vi "ZeroMQ_TCS.vi"() -> ()   [LabVIEW 2018]
uses:
  <vilib>/addons/zeromq/socket_type.ctl
  <vilib>/addons/zeromq/socket_options.ctl
  <vilib>/addons/zeromq/zeromq.lvlib
  <vilib>/addons/zeromq/zmq_socket.lvclass
  <vilib>/addons/zeromq/zmq_context.lvclass
panel:
  in  "stop 3":bool
  out "command":string
  out "error out 3":errorcluster
  out "message":string
  out "error out 2":errorcluster
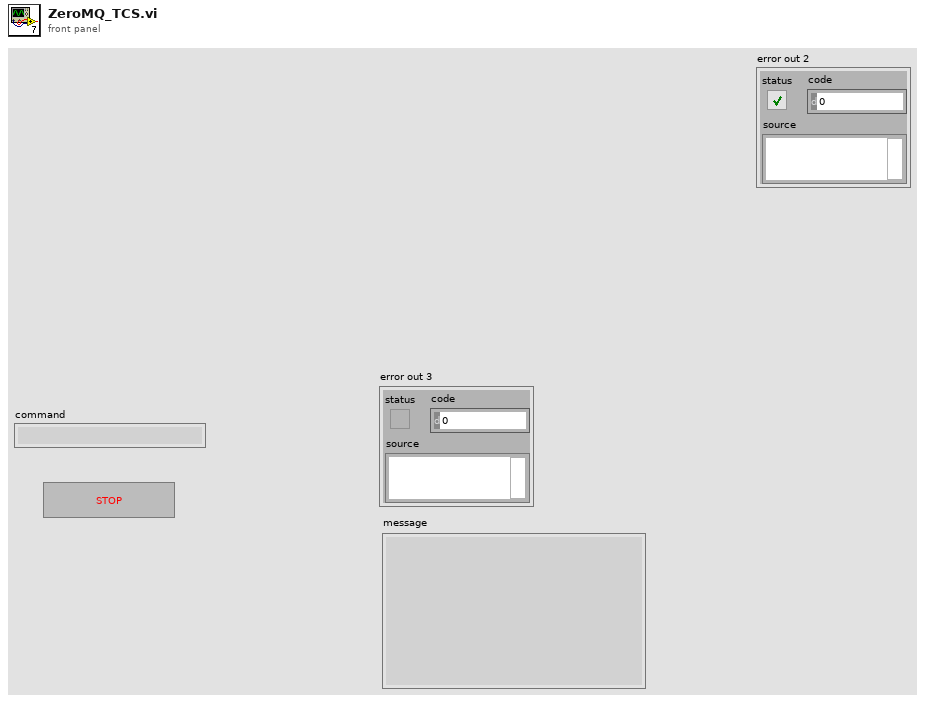
[diagram p1: front panel]
types:
  T1 = cluster{"ID":u32, "Address":string, "Service Name 1":string, "Service Name 2":string, "queue TX":refnum<queue>, "queue RX":refnum<queue>, "Port 1":u32, "Port 2":u32}
  T2 = typedef "zeromq.lvlib/socket_options.ctl" = enum8{"NONE", "ZMQ_HWM", "<2>", "ZMQ_SWAP", "ZMQ_AFFINITY", "ZMQ_ROUTING_ID", "ZMQ_SUBSCRIBE", "ZMQ_UNSUBSCRIBE", "ZMQ_RATE", "ZMQ_RECOVERY_IVL", "ZMQ_MCAST_LOOP", "ZMQ_SNDBUF", "ZMQ_RCVBUF", "ZMQ_RCVMORE", "ZMQ_FD", "ZMQ_EVENTS", "ZMQ_TYPE", "ZMQ_LINGER", "ZMQ_RECONNECT_IVL", "ZMQ_BACKLOG", "ZMQ_RECOVERY_IVL_MSEC", "ZMQ_RECONNECT_IVL_MAX", "ZMQ_MAXMSGSIZE", "ZMQ_SNDHWM", "ZMQ_RCVHWM", "ZMQ_MULTICAST_HOPS", "<26>", "ZMQ_RCVTIMEO", "ZMQ_SNDTIMEO", "<29>", "<30>", "ZMQ_IPV4ONLY", "ZMQ_LAST_ENDPOINT", "ZMQ_ROUTER_MANDATORY", "ZMQ_TCP_KEEPALIVE", "ZMQ_TCP_KEEPALIVE_CNT", "ZMQ_TCP_KEEPALIVE_IDLE", "ZMQ_TCP_KEEPALIVE_INTVL", "ZMQ_TCP_ACCEPT_FILTER", "ZMQ_IMMEDIATE", "ZMQ_XPUB_VERBOSE", "ZMQ_ROUTER_RAW", "ZMQ_IPV6", "ZMQ_MECHANISM", "ZMQ_PLAIN_SERVER", "ZMQ_PLAIN_USERNAME", "ZMQ_PLAIN_PASSWORD", "ZMQ_CURVE_SERVER", "ZMQ_CURVE_PUBLICKEY", "ZMQ_CURVE_SECRETKEY", "ZMQ_CURVE_SERVERKEY", "ZMQ_PROBE_ROUTER", "ZMQ_REQ_CORRELATE", "ZMQ_REQ_RELAXED", "ZMQ_CONFLATE", "ZMQ_ZAP_DOMAIN", "ZMQ_ROUTER_HANDOVER", "ZMQ_TOS", "ZMQ_IPC_FILTER_PID", "ZMQ_IPC_FILTER_UID", "ZMQ_IPC_FILTER_GID", "ZMQ_CONNECT_ROUTING_ID", "ZMQ_GSSAPI_SERVER", "ZMQ_GSSAPI_PRINCIPAL", "ZMQ_GSSAPI_SERVICE_PRINCIPAL", "ZMQ_GSSAPI_PLAINTEXT", "ZMQ_HANDSHAKE_IVL", "<67>", "ZMQ_SOCKS_PROXY", "ZMQ_XPUB_NODROP", "ZMQ_BLOCKY", "ZMQ_XPUB_MANUAL", "ZMQ_XPUB_WELCOME_MSG", "ZMQ_STREAM_NOTIFY", "ZMQ_INVERT_MATCHING", "ZMQ_HEARTBEAT_IVL", "ZMQ_HEARTBEAT_TTL", "ZMQ_HEARTBEAT_TIMEOUT", "ZMQ_XPUB_VERBOSER", "ZMQ_CONNECT_TIMEOUT", "ZMQ_TCP_MAXRT", "ZMQ_THREAD_SAFE", "<82>", "<83>", "ZMQ_MULTICAST_MAXTPDU", "ZMQ_VMCI_BUFFER_SIZE", "ZMQ_VMCI_BUFFER_MIN_SIZE", "ZMQ_VMCI_BUFFER_MAX_SIZE", "ZMQ_VMCI_CONNECT_TIMEOUT", "ZMQ_USE_FD", "ZMQ_GSSAPI_PRINCIPAL_NAMETYPE", "ZMQ_GSSAPI_SERVICE_PRINCIPAL_NAMETYPE", "ZMQ_BINDTODEVICE", "ZMQ_ZAP_ENFORCE_DOMAIN", "ZMQ_LOOPBACK_FASTPATH", "ZMQ_METADATA", "ZMQ_MULTICAST_LOOP", "ZMQ_ROUTER_NOTIFY"}
  T3 = typedef "zeromq.lvlib/socket_type.ctl" = enum8{"ZMQ_PAIR", "ZMQ_PUB", "ZMQ_SUB", "ZMQ_REQ", "ZMQ_REP", "ZMQ_DEALER", "ZMQ_ROUTER", "ZMQ_PULL", "ZMQ_PUSH", "ZMQ_XPUB", "ZMQ_XSUB", "ZMQ_STREAM", "ZMQ_SERVER", "ZMQ_CLIENT", "ZMQ_RADIO", "ZMQ_DISH", "ZMQ_GATHER", "ZMQ_SCATTER", "ZMQ_DGRAM"}
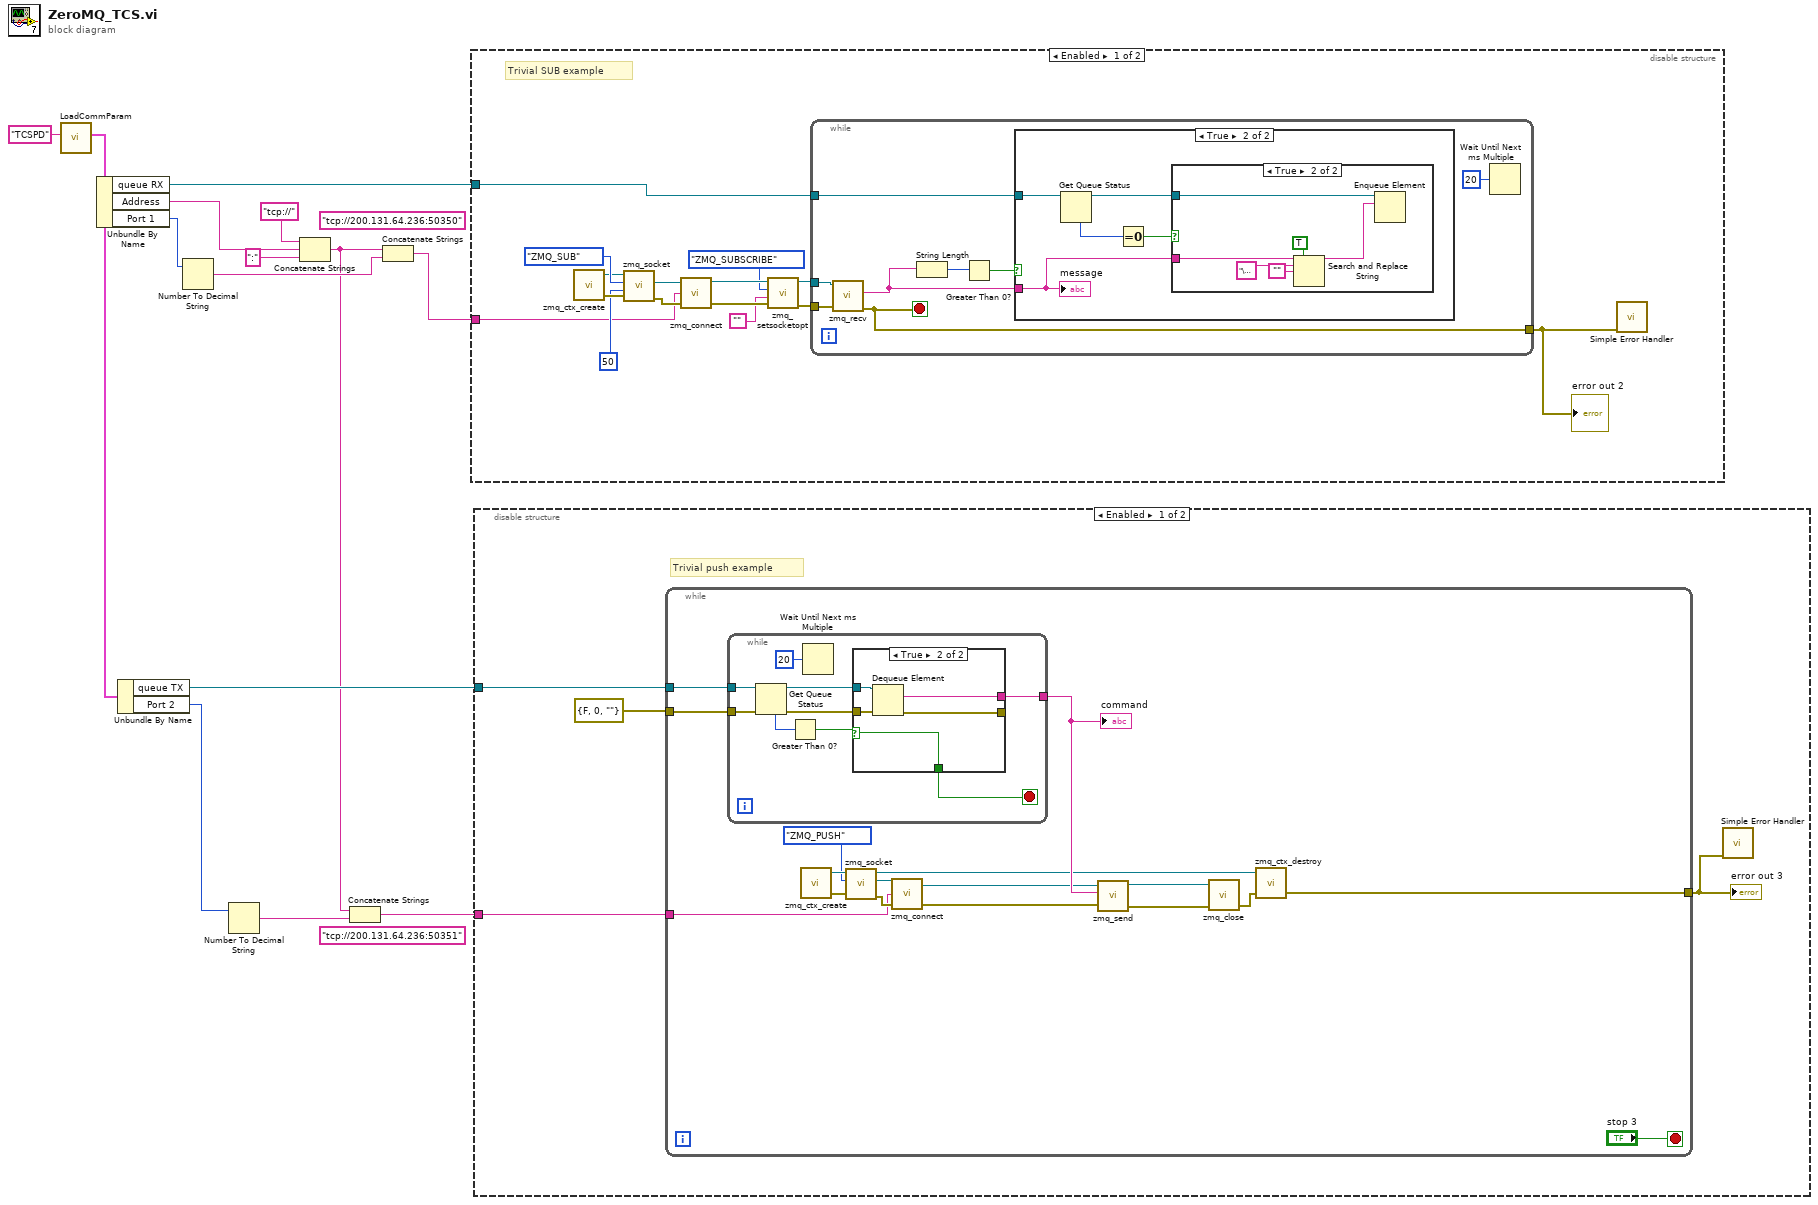
[diagram p0: block diagram]
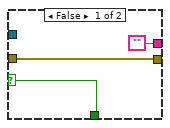
[diagram p2: hidden frame]
diagram:
  (unwired) "tcp://200.131.64.236:50351" ("endpoint")
  (unwired) "tcp://200.131.64.236:50350" ("endpoint")
  n1 = call "LoadCommParam.vi"("section name"="TCSPD") -> ("output cluster"=w7:T1)  [unwired: 10 in]
  n2 = Unbundle By Name(w7) -> ("queue RX"=w13:refnum<queue>, "Address"=w11:string, "Port 1"=w9:u32)
  n3 = Unbundle By Name(w7) -> ("queue TX"=w8:refnum<queue>, "Port 2"=w4:u32)
  n4 = Number To Decimal String(number=w9) -> (decimal integer string=w6:string)  [unwired: 1 in]
  n5 = Number To Decimal String(number=w4) -> (decimal integer string=w2:string)  [unwired: 1 in]
  n6 = Concatenate Strings("tcp://" ("string"), w11, ":" ("string")) -> (w3:string)
  n7 = Concatenate Strings(w3, w2) -> (w1:string)
  n8 = Concatenate Strings(w3, w6) -> (w5:string)
  n9 = disable-structure shown="Enabled" {
    disable-tunnel: w13 -> [w16 _]
    disable-tunnel: w5 -> [w15 _]
    frame Enabled {
      # "Trivial SUB example"
      n10 = call <vilib>:"zmq_ctx_create.vi"() -> ("error out"=w28:errorcluster, "context out"=w18:refnum<class "zmq_context.lvclass">)  [unwired: 4 in]
      n11 = call <vilib>:"zmq_socket.vi"("error in"=w28, "linger (ms)"=50, "socket type"=socket_type."ZMQ_SUB", "context in"=w18) -> ("error out"=w27:errorcluster, "socket out"=w19:refnum<class "zmq_socket.lvclass">)  [unwired: 1 in, 1 out]
      n12 = call <vilib>:"zmq_connect.vi"("error in"=w27, "endpoint"=w15, "socket in"=w19) -> ("error out"=w25:errorcluster, "socket out"=w26:refnum<class "zmq_socket.lvclass">)  [unwired: 1 in]
      n13 = call <vilib>:"zmq_setsocketopt.vi"("error in"=w25, "value"="", "option"=socket_options."ZMQ_SUBSCRIBE", "socket in"=w26) -> ("error out"=w24:errorcluster, "socket out"=w23:refnum<class "zmq_socket.lvclass">)  [unwired: 2 in]
      n14 = while {
        tunnel: w23 -> [w35]
        tunnel: w24 -> [w37]
        tunnel: [w36] -> w20
        tunnel: w16 -> [w32]
        stop <- w36 stop-if-true
        n15 = call <vilib>:"zmq_recv.vi"("error in"=w37, "socket in"=w35) -> ("error out"=w36:errorcluster, "data"=w31:string)  [unwired: 3 in, 3 out]
        n16 = String Length(string=w31) -> (length=w34:i32)
        n17 = Greater Than 0?(x=w34) -> (x > 0?=w33:bool)
        n18 = case shown="True" w33 {
          tunnel: w32 -> [_ w41]
          tunnel: w31 -> [_ w38]
          frame False {
          }
          frame True {
            n19 = Get Queue Status(queue=w41) -> (queue out=w39:refnum<queue>, # elements in queue=w42:i32)  [unwired: 2 in, 6 out]
            n20 = Equal To 0?(x=w42) -> (x = 0?=w40:bool)
            n21 = case shown="True" w40 {
              tunnel: w39 -> [_ w48]
              tunnel: w38 -> [_ w47]
              frame False {
              }
              frame True {
                n22 = Search and Replace String(replace all?=TRUE ("replace all? (F)"), input string=w47, search string="\u0000" ("substring (\"\")"), replace string="" ("replace string (\"\")")) -> (result string=w43:string)  [unwired: 4 in, 3 out]
                n23 = Enqueue Element(queue=w48, element=w43) -> ()  [unwired: 2 in, 3 out]
              }
            }
            "message" <- w38
          }
        }
        n24 = Wait Until Next ms Multiple(millisecond multiple=u32 20) -> ()  [unwired: 1 out]
      }
      "error out 2" <- w20
      n25 = call <vilib>:"Simple Error Handler.vi"("error in (no error)"=w20) -> ()  [unwired: 4 in, 5 out]
    }
    frame Disabled {
    }
  }
  n26 = disable-structure shown="Enabled" {
    disable-tunnel: w8 -> [w50 _]
    disable-tunnel: w1 -> [w49 _]
    frame Enabled {
      # "Trivial push example"
      n27 = while {
        tunnel: w50 -> [w69]
        tunnel: errorcluster {"status"=FALSE, "code"=0, "source"=""} ("error out") -> [w68]
        tunnel: [w57] -> w52
        tunnel: w49 -> [w53]
        stop <- "stop 3" stop-if-true
        n28 = while {
          tunnel: w69 -> [w77]
          tunnel: w68 -> [w76]
          tunnel: [w72] -> w67
          stop <- w71 stop-if-true
          n29 = Get Queue Status(queue=w77, error in (no error)=w76) -> (queue out=w73:refnum<queue>, error out=w74:errorcluster, # elements in queue=w78:i32)  [unwired: 1 in, 5 out]
          n30 = Greater Than 0?(x=w78) -> (x > 0?=w75:bool)
          n31 = Wait Until Next ms Multiple(millisecond multiple=u32 20) -> ()  [unwired: 1 out]
          n32 = case shown="True" w75 {
            selector: w75 -> [w79 w82]
            tunnel: w74 -> [w81 w86]
            tunnel: w73 -> [_ w85]
            tunnel: [w81 w84] -> _
            tunnel: ["" w83] -> w72
            tunnel: [w79 w82] -> w71
            frame False {
            }
            frame True {
              n33 = Dequeue Element(queue=w85, error in (no error)=w86) -> (element=w83:string, error out=w84:errorcluster)  [unwired: 1 in, 2 out]
            }
          }
        }
        "command" <- w67
        n34 = call <vilib>:"zmq_ctx_create.vi"() -> ("error out"=w62:errorcluster, "context out"=w65:refnum<class "zmq_context.lvclass">)  [unwired: 4 in]
        n35 = call <vilib>:"zmq_socket.vi"("error in"=w62, "socket type"=socket_type."ZMQ_PUSH", "context in"=w65) -> ("error out"=w64:errorcluster, "socket out"=w63:refnum<class "zmq_socket.lvclass">, "context out"=w56:refnum<class "zmq_context.lvclass">)  [unwired: 2 in]
        n36 = call <vilib>:"zmq_connect.vi"("error in"=w64, "endpoint"=w53, "socket in"=w63) -> ("error out"=w59:errorcluster, "socket out"=w60:refnum<class "zmq_socket.lvclass">)  [unwired: 1 in]
        n37 = call <vilib>:"zmq_send.vi"("error in"=w59, "data"=w67, "socket in"=w60) -> ("error out"=w54:errorcluster, "socket out"=w55:refnum<class "zmq_socket.lvclass">)  [unwired: 4 in]
        n38 = call <vilib>:"zmq_close.vi"("error in"=w54, "socket"=w55) -> ("error out"=w58:errorcluster)  [unwired: 3 in]
        n39 = call <vilib>:"zmq_ctx_destroy.vi"("error in"=w58, "context in"=w56) -> ("error out"=w57:errorcluster)  [unwired: 3 in]
      }
      "error out 3" <- w52
      n40 = call <vilib>:"Simple Error Handler.vi"("error in (no error)"=w52) -> ()  [unwired: 4 in, 5 out]
    }
    frame Disabled {
    }
  }
